vi "Scripting_FitToLargestDec.vi"(4 "error in (no error)":errorcluster, 6 "border spacing (2 px)":i32=2, 7 "VI Ref (calling VI)":refnum<vi>) -> (0 "error out":errorcluster, 3 "dup VI Ref":refnum<vi>)   [LabVIEW 2020]
doc: "This utility will fit (resize and center) a VI (defined by the \"VI Ref\" input) about the largest decoration in that VI. It will add a border defined by border spacing in units of pixels. If there are no decorations found in the VI it is a no-op and will not produce an error. Unfortunately, this VI can not find locked decorations (yet)."
panel:
  # "[OpenG VI Tags] ***Do Not Remove***\nSVN Revision = 331\nSVN Revision Date = 2007-01-07 09:51:31 -0800 (Sun, 07 Jan 2007)\nPackage = oglib_appcontrol-2.9-1\nDepends ="
  # "Fit VI window to Largest Decoration.vi\n\nFits a VI's front panel window to its largest decoration size.\n\nPlease visit http://www.OpenG.org to learn about the\nOpen Source LabVIEW software movement.\n\nNOTICE -- YOU MUST LEAVE THIS NOTICE IN PLACE.  PER THE TERMS OF THE LICENSE BELOW, YOU MAY SUBLICENSE THIS SOFTWARE \nIN ANY WAY THAT DOES NOT CONFLICT WITH THIS LICENSE.\n\n### BSD License (http://www.opensource.org/licenses/bsd-license.php) Begin ###\n \nCopyright (c) 2002, Jim Kring <jim@jimkring.com>\nCopyright (c) 2002, Cal-Bay Systems, Inc. <info@calbay.com>\n\nAll rights reserved.\n\nRedistribution and use in source and binary forms, with or without modification, are permitted provided that the following conditions are met:\n\n    * Redistributions of source code must retain the above copyright notice, this list of conditions and the following disclaimer.\n    * Redistributions in binary form must reproduce the above copyright notice, this list of conditions and the following disclaimer in the \n       documentation and/or other materials provided with the distribution.\n    * Neither the name of SciWare, James Kring, Inc., nor the names of its contributors may be used to endorse or promote products derived \n       from this software without specific prior written permission.\n\nTHIS SOFTWARE IS PROVIDED BY THE COPYRIGHT HOLDERS AND CONTRIBUTORS \"AS IS\" AND ANY EXPRESS OR IMPLIED WARRANTIES, \nINCLUDING, BUT NOT LIMITED TO, THE IMPLIED WARRANTIES OF MERCHANTABILITY AND FITNESS FOR A PARTICULAR PURPOSE ARE \nDISCLAIMED. IN NO EVENT SHALL THE COPYRIGHT OWNER OR CONTRIBUTORS BE LIABLE FOR ANY DIRECT, INDIRECT, INCIDENTAL,\n SPECIAL, EXEMPLARY, OR CONSEQUENTIAL DAMAGES (INCLUDING, BUT NOT LIMITED TO, PROCUREMENT OF SUBSTITUTE GOODS OR \nSERVICES; LOSS OF USE, DATA, OR PROFITS; OR BUSINESS INTERRUPTION) HOWEVER CAUSED AND ON ANY THEORY OF LIABILITY, \nWHETHER IN CONTRACT, STRICT LIABILITY, OR TORT (INCLUDING NEGLIGENCE OR OTHERWISE) ARISING IN ANY WAY OUT OF THE USE \nOF THIS SOFTWARE, EVEN IF ADVISED OF THE POSSIBILITY OF SUCH DAMAGE.\n\n### BSD License End ###"
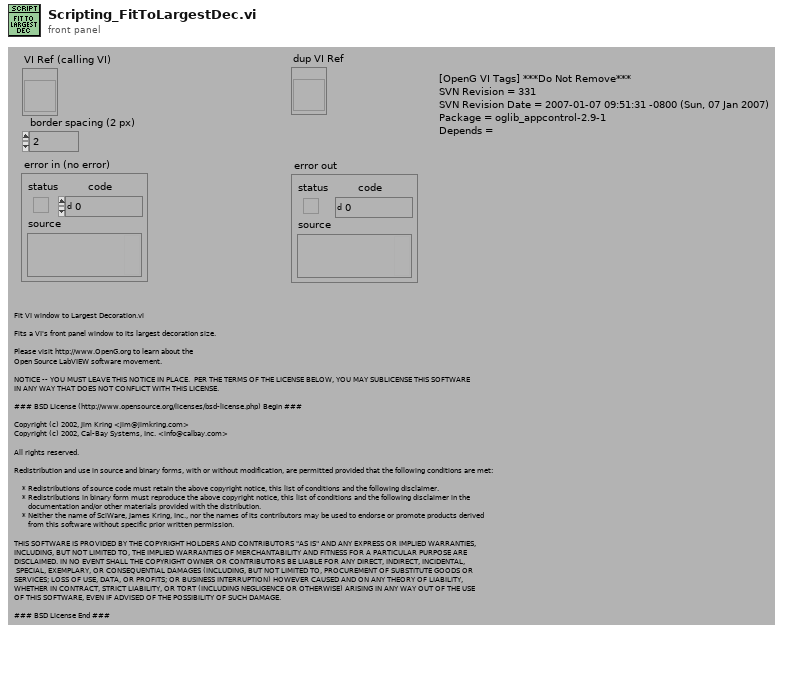
[diagram p1: front panel]
types:
  T1 = typedef "LVRectTypeDef.ctl" = cluster{"Left":i16, "Top":i16, "Right":i16, "Bottom":i16}
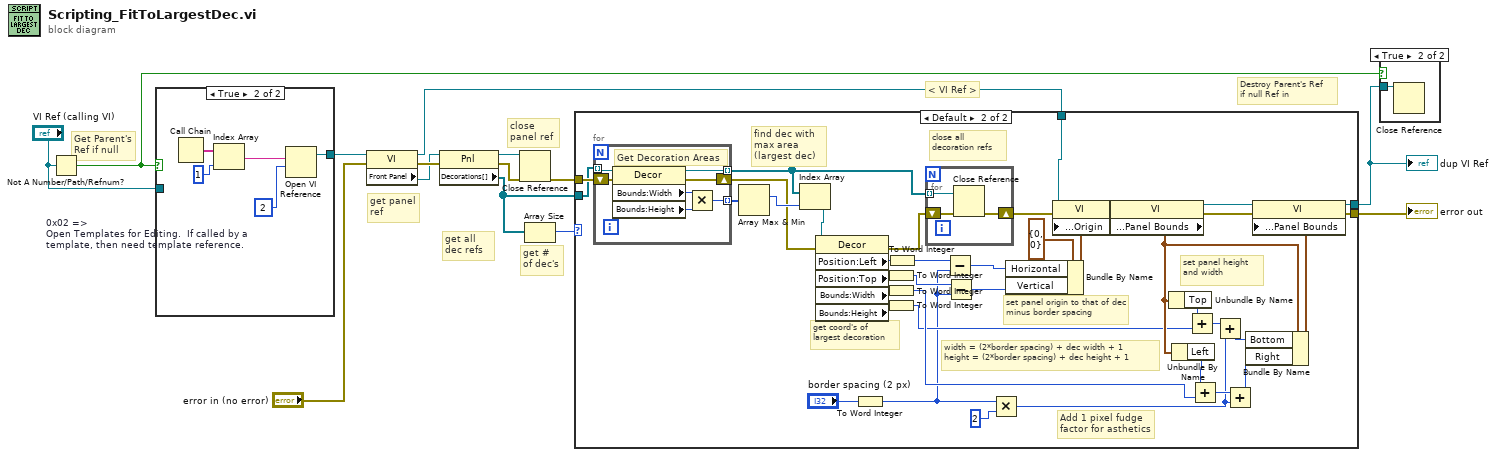
[diagram p0: block diagram]
diagram:
  # "Destroy Parent's Ref\nif null Ref in"
  # "Get Parent's\nRef if null"
  # "get # of dec's"
  # "get panel ref"
  # "get all dec refs"
  # "close panel ref"
  # "< VI Ref >"
  n1 = Not A Number/Path/Refnum?(number/path/refnum="VI Ref (calling VI)") -> (NaN/Path/Refnum?=w2:bool)
  n2 = case shown="True" w2 {
    tunnel: [w15 w16] -> w3
    tunnel: "VI Ref (calling VI)" -> [w15 _]
    frame False {
    }
    frame True {
      w17 = 2  # 0x02 => Open Templates for Editing.  If called by a template, then need template reference.
      n3 = Call Chain() -> (call chain=w20:string[])
      n4 = Index Array(array=w20, index=1 ("Index")) -> (element=w18:string)
      n5 = Open VI Reference(vi path=w18, options=w17) -> (vi reference=w16:refnum<vi>)  [unwired: 4 in, 1 out]
    }
  }
  n6 = property on="Property Node" class="VI"(reference=w3, error in="error in (no error)") -> (reference out=w14:refnum<vi>, error out=w12:errorcluster, "Front Panel"=w9:refnum<vi>)
  n7 = property on="Property Node" class="Pnl"(reference=w9, error in=w12) -> (reference out=w13:refnum<vi>, error out=w11:errorcluster, "Decorations[]"=w6:refnum<vi>[])
  n8 = Close Reference(reference=w13, error in (no error)=w11) -> (error out=w8:errorcluster)
  n9 = Array Size(array=w6) -> (size(s)=w5:i32)
  n10 = case shown="Default" w5 {
    tunnel: w14 -> [w22 w60]
    tunnel: w8 -> [w21 w43]
    tunnel: [w21 w31] -> w7
    tunnel: [w22 w30] -> w1
    tunnel: w6 -> [_ w29]
    frame 0 {
      # "do nothing if no decorations"
    }
    frame Default {
      # "width = (2*border spacing) + dec width + 1\nheight = (2*border spacing) + dec height + 1"
      # "set panel height and width"
      # "set panel origin to that of dec minus border spacing"
      # "close all  decoration refs"
      # "get coord's of largest decoration"
      # "Add 1 pixel fudge factor for asthetics"
      # "find dec with max area (largest dec)"
      n11 = for {
        tunnel: w29 -> [w69] mode=indexing
        tunnel: [w66] -> w42 mode=indexing
        shift-right: [w64] -> w38
        shift-left: w43 -> [w65]
        tunnel: [w63] -> w40 mode=indexing
        # "Get Decoration Areas"
        n12 = property class="Decor"(reference=w69, error in=w65) -> (reference out=w63:refnum<vi>, error out=w64:errorcluster, "Bounds:Width"=w68:u32, "Bounds:Height"=w67:u32)
        n13 = Multiply(x=w68, y=w67) -> (x*y=w66:u32)
      }
      n14 = Array Max & Min(array=w42) -> (max index (indices)=w41:i32)  [unwired: 3 out]
      n15 = Index Array(array=w40, index=w41) -> (element=w39:refnum<vi>)
      n16 = property class="Decor"(reference=w39, error in=w38) -> (error out=w37:errorcluster, "Position:Left"=w46:i32, "Position:Top"=w49:i32, "Bounds:Width"=w54:u32, "Bounds:Height"=w52:u32)  [unwired: 1 out]
      n17 = To Word Integer(number="border spacing (2 px)") -> (16bit integer=w23:i16)
      n18 = To Word Integer(number=w49) -> (16bit integer=w24:i16)
      n19 = To Word Integer(number=w54) -> (16bit integer=w27:i16)
      n20 = To Word Integer(number=w52) -> (16bit integer=w26:i16)
      n21 = To Word Integer(number=w46) -> (16bit integer=w25:i16)
      n22 = for {
        tunnel: w40 -> [w72] mode=indexing
        shift-right: [w70] -> w34
        shift-left: w37 -> [w71]
        n23 = Close Reference(reference=w72, error in (no error)=w71) -> (error out=w70:errorcluster)
      }
      n24 = Subtract(x=w25, y=w23) -> (x-y=w47:i16)
      n25 = Subtract(x=w24, y=w23) -> (x-y=w48:i16)
      n26 = Multiply(x=w23, y=i16 2) -> (x*y=w28:i16)
      n27 = Bundle By Name(cluster=cluster{"Horizontal":i16, "Vertical":i16} {"Horizontal"=0, "Vertical"=0} ("Front Panel Window:Origin"), "Horizontal"=w47, "Vertical"=w48) -> (w44:cluster{"Horizontal":i16, "Vertical":i16})
      n28 = property on="Property Node" class="VI"(reference=w60, error in=w34, "Front Panel Window:Origin"=w44) -> (reference out=w61:refnum<vi>, error out=w33:errorcluster)
      n29 = property on="Property Node" class="VI"(reference=w61, error in=w33) -> (reference out=w62:refnum<vi>, error out=w32:errorcluster, "Front Panel Window:Panel Bounds"=w50:T1)
      n30 = Unbundle By Name(w50) -> ("Top"=w51:i16)
      n31 = Unbundle By Name(w50) -> ("Left"=w53:i16)
      n32 = Add(x=w51, y=w26) -> (x+y=w58:i16)
      n33 = Add(x=w53, y=w27) -> (x+y=w56:i16)
      n34 = Add(x=w58, y=w28) -> (x+y=w59:i16)
      n35 = Add(x=w56, y=w28) -> (x+y=w57:i16)
      n36 = Bundle By Name(cluster=w50, "Bottom"=w59, "Right"=w57) -> (w55:T1)
      n37 = property on="Property Node" class="VI"(reference=w62, error in=w32, "Front Panel Window:Panel Bounds"=w55) -> (reference out=w30:refnum<vi>, error out=w31:errorcluster)
    }
  }
  "error out" <- w7
  "dup VI Ref" <- w1
  n38 = case shown="True" w2 {
    tunnel: w1 -> [_ w73]
    frame False {
    }
    frame True {
      n39 = Close Reference(reference=w73) -> ()  [unwired: 1 in, 1 out]
    }
  }
